vi "URI.vi"(11 "IErrorHandler in":refnum<class "IErrorHandler.lvclass">) -> (2 "URI":string, 3 "IErrorHandler out":refnum<class "IErrorHandler.lvclass">)   [LabVIEW 2020, in "wamplv.lvlib" / "IAbortOrErrorHandler.lvclass"]
uses:
  Error/IAbortOrErroHandler/IAbortOrErrorHandler.lvclass
  IErrorHandler.lvclass
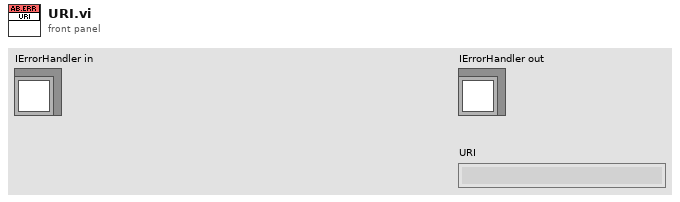
[diagram p1: front panel]
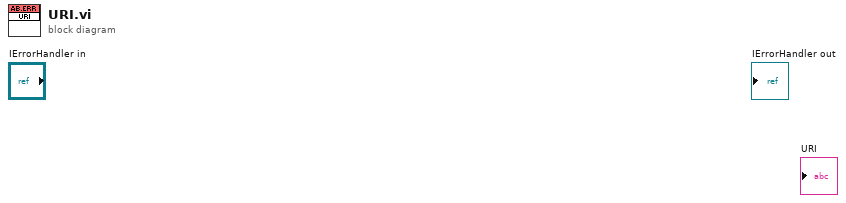
[diagram p0: block diagram]
diagram:
